vi "ScratchTest.vi"() -> ()   [LabVIEW 2014]
panel:
  out "x < y?":bool
  in  "stop":bool
  out "lo(x) 3":u8
  out "hi(x) 3":u8
  out "lo(x) 2":u8
  out "hi(x) 2":u8
  out "unsigned 32bit integer":u32
  out "lo(x)":u8
  out "hi(x)":u8
  in  "U16":u16
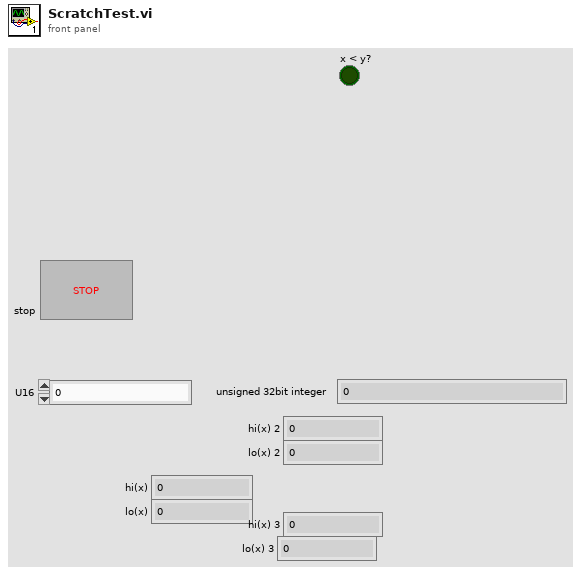
[diagram p1: front panel]
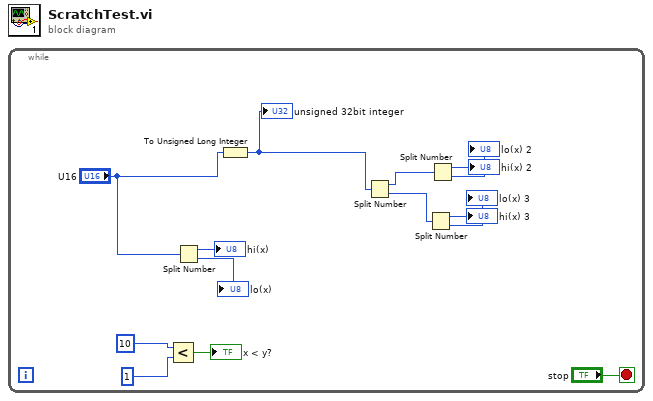
[diagram p0: block diagram]
diagram:
  n1 = while {
    stop <- "stop" stop-if-true
    n2 = Less?(x=u32 10, y=u32 1 ("x")) -> (x < y?=→"x < y?":bool)
    n3 = Split Number(x="U16") -> (hi(x)=→"hi(x)":u8, lo(x)=→"lo(x)":u8)
    n4 = To Unsigned Long Integer(number="U16") -> (unsigned 32bit integer=w11:u32)
    "unsigned 32bit integer" <- w11
    n5 = Split Number(x=w11) -> (hi(x)=w10:u16, lo(x)=w9:u16)
    n6 = Split Number(x=w9) -> (hi(x)=→"hi(x) 3":u8, lo(x)=→"lo(x) 3":u8)
    n7 = Split Number(x=w10) -> (hi(x)=→"hi(x) 2":u8, lo(x)=→"lo(x) 2":u8)
  }
